vi "DepthSense Recorder.vi"() -> ()   [LabVIEW 2011]
uses:
  <vilib>/Utility/sysdir.llb/System Directory Type.ctl
  DepthSense/IT WORKS SO SUCK IT/DepthSense Global Status.vi
  <vilib>/vision/NI_Vision_Development_Module.lvlib
panel:
  in  "stop 2":bool
  out "Image 2":T1(plugin-control)
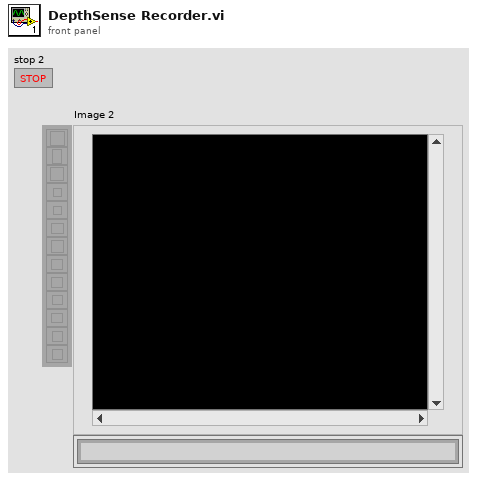
[diagram p1: front panel]
types:
  T1 = typedef "IMAQ Image.ctl" = refnum<image>
  T2 = typedef "System Directory Type.ctl" = i32
  T3 = typedef "t_CallbackReferences.ctl" = cluster{"LV event callback ":refnum<k27>, "Proxy instance":refnum<k24>, "(*f)(...)":i32}
  T4 = typedef "Image Type" = u32
  T5 = cluster{"Camera Version":string, "Image Height":i32, "Image Width":i32, "Minimum Framerate":i32, "Maximum Framerate":i32, "Framerate":i32, "Close Mode":bool, "Denoising":bool, "Leakage Algorithm":bool, "Anti-Aliasing":bool, "Camera Status":i32, "API Version":string, "Light Intensity":i32, "Confidence Threshold":u16, "Range":sgl}
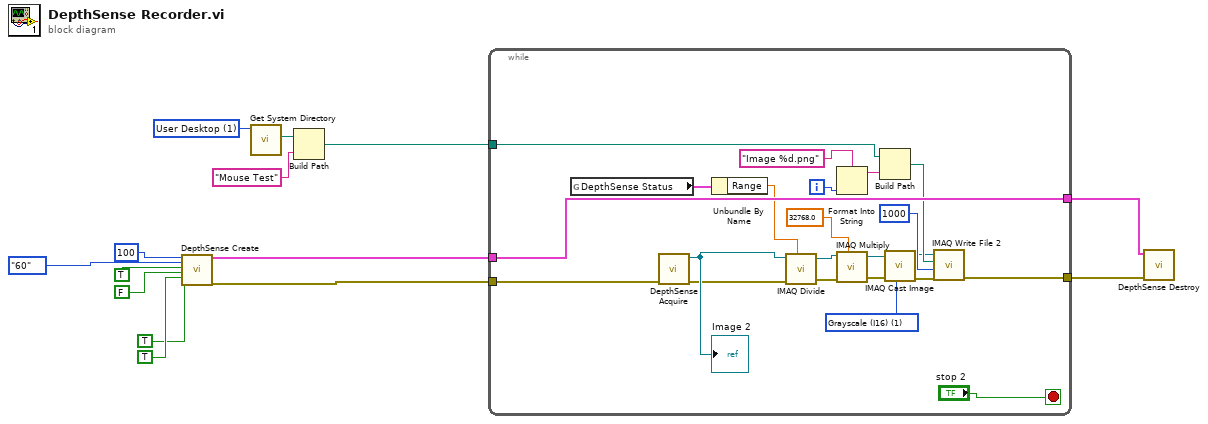
[diagram p0: block diagram]
diagram:
  w14 = T2 1 items=["User Home"=0, "User Desktop"=1, "User Documents"=2, "User Application Data"=3, "User Preferences"=4, "User Temporary"=5, "Public Documents"=6, "Public Application Data"=7, "Public Preferences"=8, "Public Cache"=13, "System Core Libraries"=9, "System Installed Libraries"=10, "Application Files"=11, "Boot Volume Root"=12] ("system directory type")
  n1 = call "DepthSense Create.vi"("Confidence"=100, "Framerate"=enum32{"25", "30", "50", "60"}."60", "Close Mode?"=TRUE, "Denoise?"=FALSE, "Anti-Alias?"=TRUE, "Correct Leakage?"=TRUE) -> ("callbacks"=w10:cluster{"References":T3, "References":T3}, "error out"=w11:errorcluster)  [unwired: 11 in, 1 out]
  n2 = call <vilib>:"Get System Directory.vi"("system directory type"=w14) -> ("system directory"=w13:path)  [unwired: 10 in]
  n3 = Build Path(base path=w13, name or relative path="Mouse Test") -> (appended path=w4:path)
  n4 = while {
    tunnel: w11 -> [w36]
    tunnel: [w23] -> w5
    tunnel: [w34] -> w9
    tunnel: w10 -> [w34]
    tunnel: w4 -> [w26]
    i -> [w24]
    stop <- "stop 2" stop-if-true
    w16 = T4 1 items=["Grayscale (U8)", "Grayscale (I16)", "Grayscale (SGL)", "Complex (CSG)", "RGB (U32)", "HSL (U32)", "RGB (U64)", "Grayscale (U16)"] ("Image Type")
    n5 = global read "DepthSense Global Status.vi" "DepthSense Status"() -> (w33:T5)
    n6 = call "DepthSense Acquire.vi"("error in (no error)"=w36) -> ("error out"=w15:errorcluster, "new depth frame"=w28:T1)  [unwired: 9 in]
    "Image 2" <- w28
    n7 = Unbundle By Name(w33) -> ("Range"=w32:sgl)
    n8 = call "IMAQ Divide"("Image Src A"=w28, "Constant"=w32, "error in (no error)"=w15) -> ("Image Dst Out"=w30:T1, "error out"=w31:errorcluster)  [unwired: 4 in]
    n9 = Format Into String(format string="Image %d.png", w24) -> (resulting string=w25:string)  [unwired: 2 in, 1 out]
    n10 = call "IMAQ Multiply"("Image Src A"=w30, "Constant"=sgl 32768.0, "error in (no error)"=w31) -> ("Image Dst Out"=w17:T1, "error out"=w20:errorcluster)  [unwired: 4 in]
    n11 = Build Path(base path=w26, name or relative path=w25) -> (appended path=w22:path)
    n12 = call "IMAQ Cast Image"("Image Type"=w16, "error in (no error)"=w20, "Image Src"=w17) -> ("error out"=w19:errorcluster, "Image Dst Out"=w18:T1)  [unwired: 7 in]
    n13 = call-poly "IMAQ Write File 2"("error in (no error)"=w19, "Image Quality"=u32 1000, "File Path"=w22, "Image"=w18) -> ("error out"=w23:errorcluster)  [unwired: 6 in, 1 out]
  }
  n14 = call "DepthSense Destroy.vi"("error in (no error)"=w5, "callbacks"=w9) -> ()  [unwired: 9 in, 1 out]
